vi "Nominal Core Streaming.Async.vi"(10 "Parameters":variant, 11 "Process":refnum<class "Process.lvclass">) -> ()   [LabVIEW 2026, in "Nominal Core Streaming Engine.lvlib"]
uses:
  Nominal Core Streaming Engine.lvlib
  <vilib>/NI/NIVS Inline Async API/_VS Inline Async API/Process/Process.lvclass
  rt full channel buffer.ctl
  rt per channel buffer.ctl
  Shared/compiled stream data.ctl
  Shared/stream configuration mode.ctl
  Shared/time convert type.ctl
  <vilib>/NI/NIVS Inline Async API/_VS Inline Async API/Process/Process.lvclass/Process.ctl
  <vilib>/NI/NIVS Inline Async API/_Data Access Engine/Access Type Classes/Read/Read.lvclass/Read.ctl
  <vilib>/NI/NIVS Inline Async API/_Data Access Engine/Access Type Classes/Write/Write.lvclass/Write.ctl
  <vilib>/NI/NIVS Inline Async API/_Data Access Engine/Data Access Engine/Methods/Read.Data.vi
  <vilib>/NI/NIVS Inline Async API/_Data Access Engine/Data Access Engine/Methods/Write.Data.vi
  <vilib>/NI/NIVS Inline Async API/_VS Inline Async API/Process/Data Member Access/Read Data Access.vi
  <vilib>/NI/NIVS Inline Async API/_VS Inline Async API/Error Handling Process/SubVIs/Error.ConvertArray.vi
  <vilib>/NI/NIVS Inline Async API/_Data Access Engine/Access Type Classes/Read/Read.ProcessData.vi
  <vilib>/NI/NIVS Inline Async API/_Data Access Engine/Access Type Classes/Write/Write.ProcessData.vi
  <vilib>/NI/NIVS Inline Async API/_Data Access Engine/Access Type Classes/Write/Write.Buffer.vi
  <vilib>/NI/NIVS Inline Async API/_Data Access Engine/Access Type Classes/Write/Write.Commit.vi
  <vilib>/NI/NIVS Inline Async API/_Data Access Engine/Data Access Engine/Methods/Write.Lookup.vi
  <vilib>/NI/NIVS Inline Async API/_Data Access Engine/Data Access Engine/Methods/Read.Lookup.vi
  <vilib>/NI/NIVS Inline Async API/_Data Access Engine/Data Access Engine/Data Access Engine.lvclass
  Shared/Nominal Core Streaming Shared.lvlib
panel:
  out "decimation":i32
  out "enabled":bool
  in  "status":i32
  out "error out":errorcluster
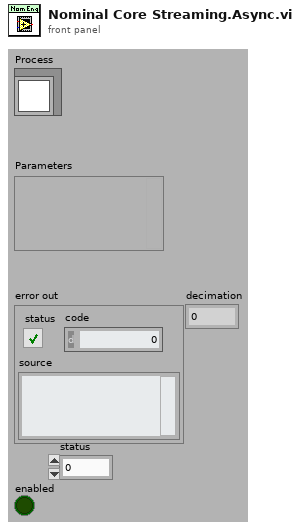
[diagram p1: front panel]
types:
  T1 = typedef "Nominal Core Streaming Engine.lvlib/rt full channel buffer.ctl" = cluster{"timestamps_ns":i64[], "per channel buffer":T2[]}
  T2 = typedef "Nominal Core Streaming Engine.lvlib/rt per channel buffer.ctl" = cluster{"Channel":u64, "values":dbl[]}
  T3 = typedef "Nominal Core Streaming Shared.lvlib/compiled stream data.ctl" = cluster{"stream name":string, "Base URL":string, "api key":string, "identifier selection":T4, "asset ID":string, "dataset name":string, "dataset ID":string, "associated channels":cluster{"Name":string, "Path":string}[], "fallback avro path":path, "time source":T5, "buffer size":u32}
  T4 = typedef "Nominal Core Streaming Shared.lvlib/stream configuration mode.ctl" = enum16{"Asset Identifier and Dataset Name", "Dataset Identifier"}
  T5 = typedef "Nominal Core Streaming Shared.lvlib/time convert type.ctl" = enum16{"to timestamp", "relative seconds"}
  T6 = typedef "Nominal Core Streaming Engine.lvlib/nominal runtime state.ctl" = cluster{"Stream":u64, "Channels":u64[], "time source":T5, "t0":timestamp}
  T7 = typedef "Data Access Engine.lvlib/Data Access Engine.lvclass/Write.DVR.ctl" = refnum<data-value>
  T8 = typedef "Data Access Engine.lvlib/Data Access Engine.lvclass/Read.DVR.ctl" = refnum<data-value>
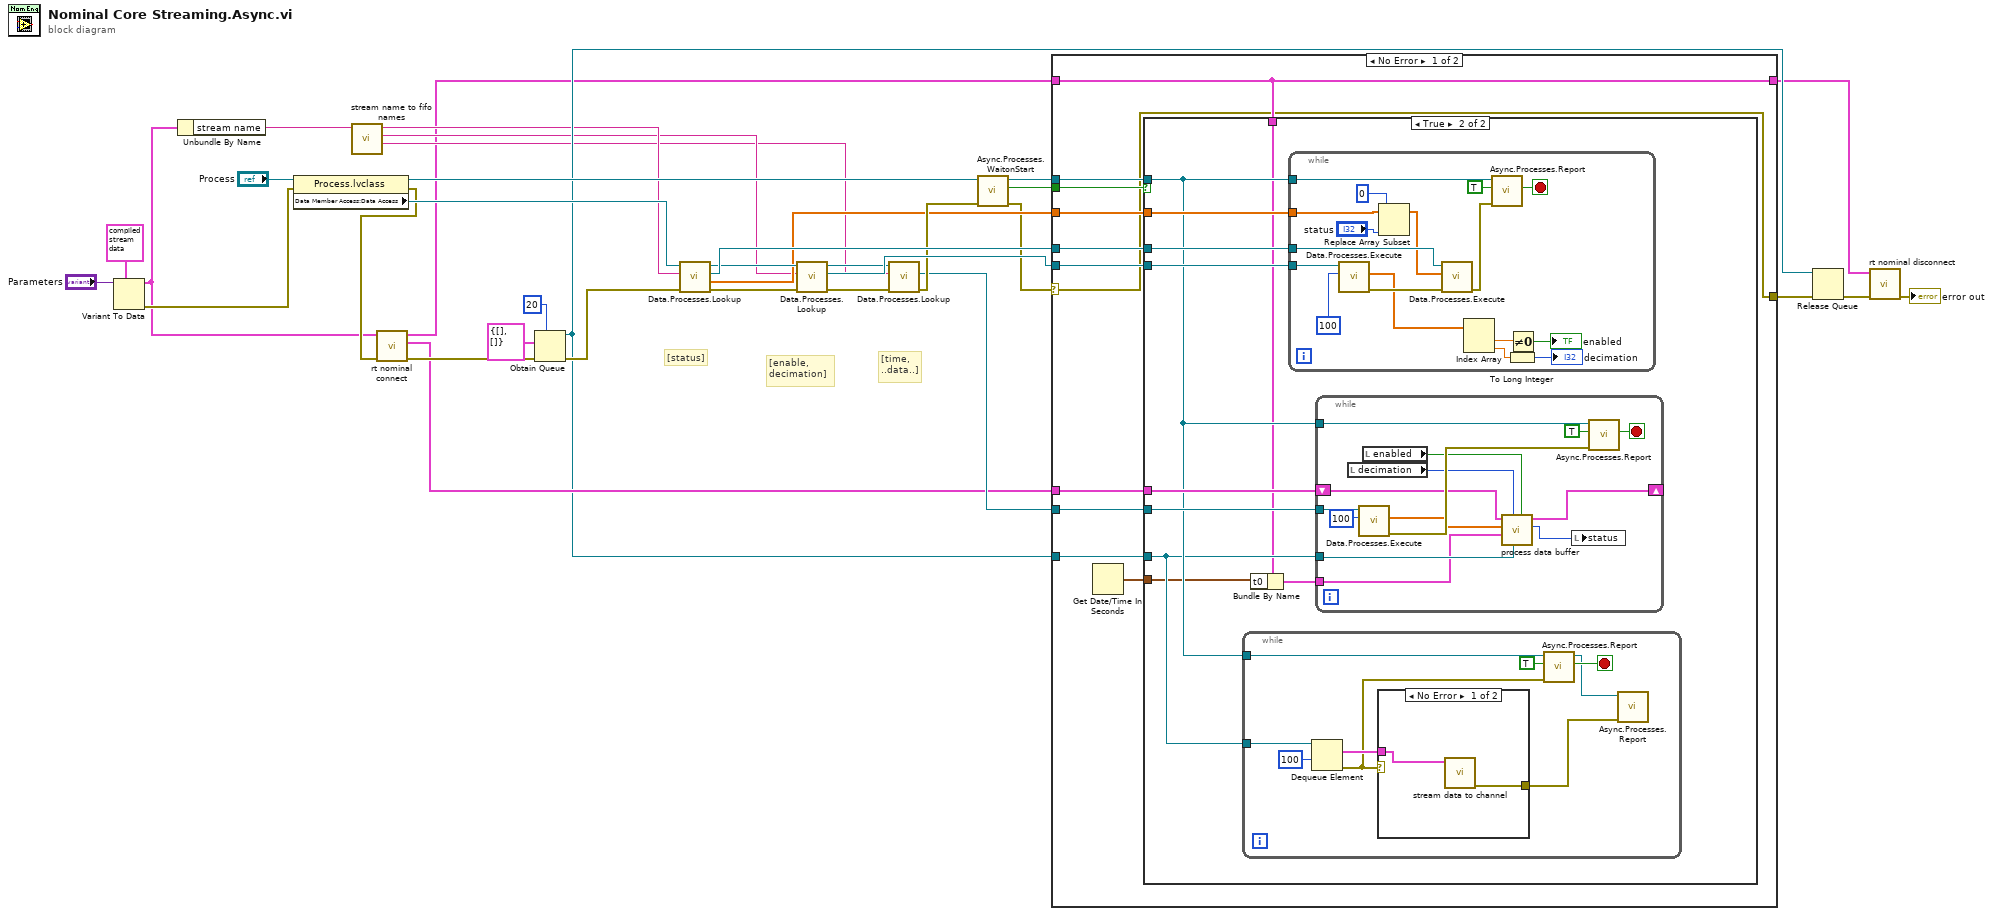
[diagram p0: block diagram]
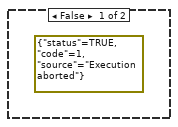
[diagram p2: hidden frame]
diagram:
  # "[time,\n..data..]"
  # "[status]"
  # "[enable,\ndecimation]"
  n1 = Variant To Data(type=T3 {"stream name"="", "Base URL"="https://api.gov.nominal.io/api/", "api key"="", "identifier selection"=enum."Asset Identifier and Dataset Name", "asset ID"="", "dataset name"="", "dataset ID"="", "associated channels"=[], "fallback avro path"=path "", "time source"=enum."to timestamp", "buffer size"=0} ("Cluster"), Variant="Parameters") -> (data=w4:T3, error out=w24:errorcluster)  [unwired: 1 in]
  n2 = Unbundle By Name(w4) -> ("stream name"=w1:string)
  n3 = property class="Process.lvclass"(reference="Process", error in=w24) -> (reference out=w28:refnum<class "Process.lvclass">, error out=w19:errorcluster, "Data Member Access:Data Access"=w27:refnum<class "Data Access Engine.lvclass">)
  n4 = call "stream name to fifo names.vi"("Name"=w1) -> ("data to CD"=w5:string, "meta to CD"=w6:string, "meta from CD"=w7:string)  [unwired: 8 in]
  n5 = call "rt nominal connect.vi"("error in"=w19, "stream configuration"=w4) -> ("error out"=w18:errorcluster, "channel buffer"=w15:T1, "nominal state"=w3:T6)  [unwired: 7 in]
  n6 = Obtain Queue(max queue size (-1, unlimited)=20, element data type=T1 {"timestamps_ns"=[], "per channel buffer"=[]} ("output cluster"), error in (no error)=w18) -> (queue out=w9:refnum<queue>, error out=w13:errorcluster)  [unwired: 2 in, 1 out]
  n7 = call-poly <vilib>:"Data.Processes.Lookup.vi"("error in (no error)"=w13, "Name"=w7, "Data Access API in"=w27) -> ("error out"=w32:errorcluster, "Initial Values"=w14:dbl[], "Ref"=w31:T7, "Data Access API out"=w30:refnum<class "Data Access Engine.lvclass">)  [unwired: 5 in]
  n8 = call-poly <vilib>:"Data.Processes.Lookup.vi"("error in (no error)"=w32, "Name"=w6, "Data Access API in"=w30) -> ("error out"=w22:errorcluster, "Ref"=w33:T8, "Data Access API out"=w23:refnum<class "Data Access Engine.lvclass">)  [unwired: 5 in, 1 out]
  n9 = call-poly <vilib>:"Data.Processes.Lookup.vi"("error in (no error)"=w22, "Name"=w5, "Data Access API in"=w23) -> ("error out"=w21:errorcluster, "Ref"=w20:T8)  [unwired: 5 in, 2 out]
  n10 = call <vilib>:"Async.Processes.WaitonStart.vi"("error in (no error)"=w21, "Process"=w28) -> ("error out"=w2:errorcluster, "Execute"=w35:bool, "Process out"=w34:refnum<class "Process.lvclass">)  [unwired: 7 in]
  n11 = case shown="No Error" w2 {
    selector: w2 -> [w37 w99]
    tunnel: w35 -> [w46 _]
    tunnel: w34 -> [w45 _]
    tunnel: w31 -> [w44 _]
    tunnel: w33 -> [w43 _]
    tunnel: w20 -> [w42 _]
    tunnel: [w41 w100] -> w8
    tunnel: w3 -> [w41 w100]
    tunnel: [w37 w99] -> w17
    tunnel: w15 -> [w40 _]
    tunnel: w14 -> [w39 _]
    tunnel: w9 -> [w38 _]
    frame No Error {
      n12 = Get Date/Time In Seconds() -> (seconds since 1Jan1904=w36:timestamp)
      n13 = case shown="True" w46 {
        tunnel: w45 -> [_ w51]
        tunnel: w43 -> [_ w56]
        tunnel: w44 -> [_ w55]
        tunnel: w42 -> [_ w54]
        tunnel: w41 -> [_ w49]
        tunnel: w40 -> [_ w53]
        tunnel: w39 -> [_ w52]
        tunnel: w38 -> [_ w50]
        tunnel: w36 -> [_ w48]
        frame False {
          (unwired) errorcluster {"status"=TRUE, "code"=1, "source"="Execution aborted"} ("error IO")
        }
        frame True {
          n14 = while {
            tunnel: w51 -> [w65]
            tunnel: w50 -> [w63]
            stop <- w64 stop-if-true
            n15 = Dequeue Element(queue=w63, timeout in ms (-1)=100) -> (element=w61:T1, error out=w58:errorcluster)  [unwired: 1 in, 2 out]
            n16 = case shown="No Error" w58 {
              tunnel: w61 -> [w67 _]
              tunnel: [w66 _] -> w57
              frame No Error {
                n17 = call "stream data to channel.vi"("data chunk"=w67) -> ("error out"=w66:errorcluster)  [unwired: 10 in]
              }
              frame Error {
              }
            }
            n18 = call <vilib>:"Async.Processes.Report.vi"("Error"=w58, "Stop Async on Error?"=TRUE, "Process in"=w65) -> ("Stop"=w64:bool, "Process out"=w59:refnum<class "Process.lvclass">)  [unwired: 7 in]
            n19 = call <vilib>:"Async.Processes.Report.vi"("Error"=w57, "Process in"=w59) -> ()  [unwired: 8 in, 2 out]
          }
          n20 = Bundle By Name(cluster=w49, "t0"=w48) -> (w47:T6)
          n21 = while {
            tunnel: w51 -> [w98]
            tunnel: w56 -> [w96]
            tunnel: w55 -> [w95]
            tunnel: w52 -> [w89]
            stop <- w97 stop-if-true
            n22 = call-poly <vilib>:"Data.Processes.Execute.vi"("timeout ms"=100, "Ref"=w96) -> ("error out"=w93:errorcluster, "Values"=w87:dbl[])  [unwired: 7 in, 1 out]
            n23 = Replace Array Subset(array=w89, new element="status", index=0) -> (w88:dbl[])
            n24 = call-poly <vilib>:"Data.Processes.Execute.vi"("error in (no error)"=w93, "Values"=w88, "Ref"=w95) -> ("error out"=w92:errorcluster)  [unwired: 8 in]
            n25 = Index Array(array=w87) -> (element #1=w86:dbl, element #2=w84:dbl)  [unwired: 2 in]
            n26 = call <vilib>:"Async.Processes.Report.vi"("Error"=w92, "Stop Async on Error?"=TRUE, "Process in"=w98) -> ("Stop"=w97:bool)  [unwired: 7 in, 1 out]
            n27 = To Long Integer(number=w84) -> (32bit integer=→"decimation":i32)
            n28 = Not Equal To 0?(x=w86) -> (x != 0?=→"enabled":bool)
          }
          n29 = while {
            tunnel: w51 -> [w81]
            tunnel: w54 -> [w77]
            shift-right: [w76] -> _
            shift-left: w53 -> [w73]
            tunnel: w50 -> [w70]
            tunnel: w47 -> [w68]
            stop <- w80 stop-if-true
            n30 = local read "decimation"() -> (w75:i32)
            n31 = call-poly <vilib>:"Data.Processes.Execute.vi"("timeout ms"=100, "Ref"=w77) -> ("error out"=w78:errorcluster, "Values"=w72:dbl[])  [unwired: 7 in, 1 out]
            n32 = local read "enabled"() -> (w74:bool)
            n33 = call "process data buffer.vi"("enabled"=w74, "completed packet queue"=w70, "decimation"=w75, "nominal state"=w68, "Values"=w72, "channel data in"=w73) -> ("lost buffers"=w71:i32, "channel data out"=w76:T1)  [unwired: 4 in]
            n34 = local write "status"(w71) -> ()
            n35 = call <vilib>:"Async.Processes.Report.vi"("Error"=w78, "Stop Async on Error?"=TRUE, "Process in"=w81) -> ("Stop"=w80:bool)  [unwired: 7 in, 1 out]
          }
        }
      }
    }
    frame Error {
    }
  }
  n36 = Release Queue(queue=w9, error in (no error)=w17) -> (error out=w10:errorcluster)  [unwired: 1 in, 2 out]
  n37 = call "rt nominal disconnect.vi"("error in"=w10, "nominal state"=w8) -> ("error out"=→"error out":errorcluster)  [unwired: 9 in]
